vi "Construct FQN.vi"(7 "Delimiter":refnum<class "Delimiter.lvclass">, 10 "Name":string, 11 "Parent FQN":string) -> (2 "FQN":string)   [LabVIEW 2014, in "UniqueName.lvlib" / "UniqueName.lvclass"]
uses:
  UniqueName.lvclass
  Delimiter/Delimiter.lvclass
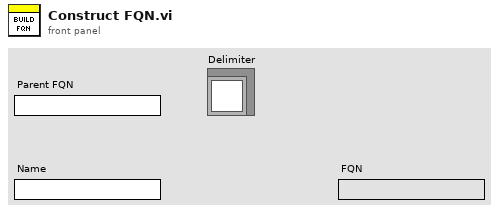
[diagram p1: front panel]
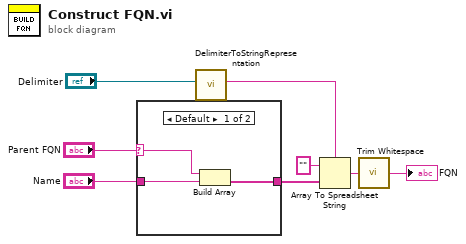
[diagram p0: block diagram]
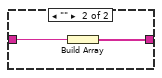
[diagram p2: hidden frame]
diagram:
  n1 = case shown="Default" "Parent FQN" {
    selector: "Parent FQN" -> [w9 _]
    tunnel: "Name" -> [w11 w13]
    tunnel: [w10 w12] -> w6
    frame Default {
      n2 = Build Array(w9, w11) -> (w10:string[])
    }
    frame "" {
      n3 = Build Array(w13) -> (w12:string[])
    }
  }
  n4 = call "DelimiterToStringRepresentation.vi"("Delimiter"="Delimiter") -> ("String representation"=w3:string)  [unwired: 10 in]
  n5 = Array To Spreadsheet String(delimiter (Tab)=w3, array=w6, 3:"" ("format string")) -> (spreadsheet string=w2:string)
  n6 = call <vilib>:"Trim Whitespace.vi"("string"=w2) -> ("trimmed string"=→"FQN":string)  [unwired: 1 in]
